vi "Acquisition_2Channels_ReceiveExternalTrigger_RisingEdge_LoggingValuesOnFile.vi"() -> ()   [LabVIEW 2018]
uses:
  <vilib>/DAQmx/read.llb/DAQmx Read (Analog 1D Wfm NChan NSamp).vi
  <vilib>/DAQmx/create/channels.llb/DAQmx Create Channel (AI-Voltage-Basic).vi
  <vilib>/DAQmx/configure/timing.llb/DAQmx Timing (Sample Clock).vi
  <vilib>/DAQmx/configure/trigger.llb/DAQmx Start Trigger (Digital Edge).vi
  <vilib>/DAQmx/miscellaneous.llb/DAQmx Fill In Error Info.vi
panel:
  in  "stop":bool
  out "Waveform Graph":waveform(dbl)[](graph)
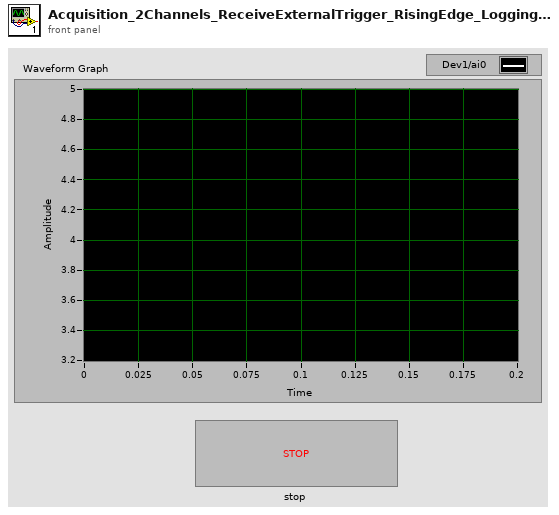
[diagram p1: front panel]
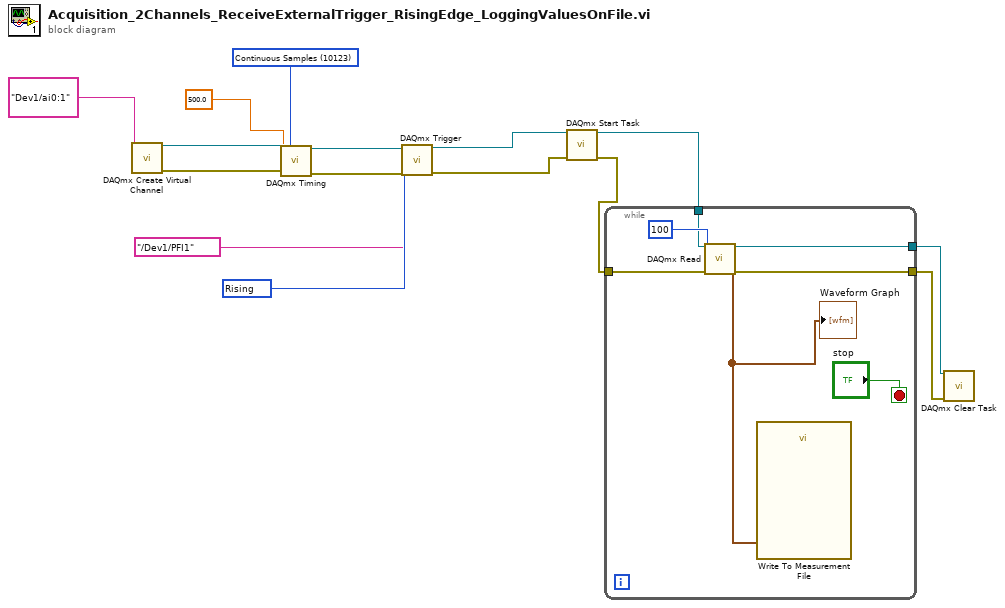
[diagram p0: block diagram]
diagram:
  w8 = 10280 items=["Rising"=10280, "Falling"=10171] ("slope")
  w12 = 10123 items=["Finite Samples"=10178, "Continuous Samples"=10123, "Hardware Timed Single Point"=12522] ("sample mode")
  n1 = call-poly <vilib>:"DAQmx Create Virtual Channel.vi"("physical channels"=tag "Dev1/ai0:1") -> ("task out"=w15:refnum<k21>, "error out"=w14:errorcluster)  [unwired: 13 in]
  n2 = call-poly <vilib>:"DAQmx Timing.vi"("task/channels in"=w15, "sample mode"=w12, "rate"=500.0, "error in"=w14) -> ("task out"=w2:refnum<k21>, "error out"=w3:errorcluster)  [unwired: 10 in]
  n3 = call-poly <vilib>:"DAQmx Trigger.vi"("task/channels in"=w2, "source"=tag "/Dev1/PFI1", "edge"=w8, "error in"=w3) -> ("task out"=w4:refnum<k21>, "error out"=w5:errorcluster)  [unwired: 10 in]
  n4 = call <vilib>:"DAQmx Start Task.vi"("task/channels in"=w4, "error in"=w5) -> ("task out"=w7:refnum<k21>, "error out"=w6:errorcluster)  [unwired: 12 in]
  n5 = while {
    tunnel: w6 -> [w21]
    tunnel: w7 -> [w20]
    tunnel: [w18] -> w10
    tunnel: [w17] -> w9
    stop <- "stop" stop-if-true
    n6 = call-poly <vilib>:"DAQmx Read.vi"("task/channels in"=w20, "number of samples per channel"=100, "error in"=w21) -> ("task out"=w18:refnum<k21>, "data"=w16:waveform(dbl)[], "error out"=w17:errorcluster)  [unwired: 10 in]
    "Waveform Graph" <- w16
    n7 = call "Write To Measurement File"("Signals"=w16) -> ()  [unwired: 16 in, 3 out]
  }
  n8 = call <vilib>:"DAQmx Clear Task.vi"("task in"=w10, "error in"=w9) -> ()  [unwired: 13 in, 1 out]
